vi "Configure Standard Waveform.vi"(8 "error in (no error)":errorcluster, 10 "Std Waveform Setting":T1={"Waveform Function (1: Sine)"=1, "Frequency (1000 Hz)"=1000.0, "Amplitude (1)"=1.0, "Unit (0: Vpp)"=0, "DC Offset (0.00 V)"=0.0} {"Unit (0: Vpp)" items=["Vpp", "Vrms", "dB"]; "Waveform Function (1: Sine)" items=["DC", "Sine", "Square", "Triangle", "Ramp", "Pulse", "Noise", "Sinc", "Negative Ramp", "Exponential Rise", "Exponential Fall", "Cardiac"]}, 11 "Abstract in":refnum<class "Abstract.lvclass">) -> (0 "error out":errorcluster, 3 "Abstract out":refnum<class "Abstract.lvclass">)   [LabVIEW 2016, in "Func Generator.lvlib" / "Abstract.lvclass"]
uses:
  Abstract.lvclass
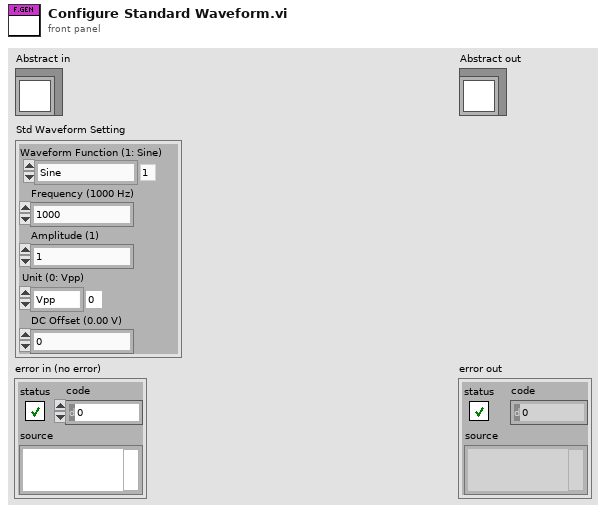
[diagram p1: front panel]
types:
  T1 = cluster{"Waveform Function (1: Sine)":u16, "Frequency (1000 Hz)":dbl, "Amplitude (1)":dbl, "Unit (0: Vpp)":u16, "DC Offset (0.00 V)":dbl}
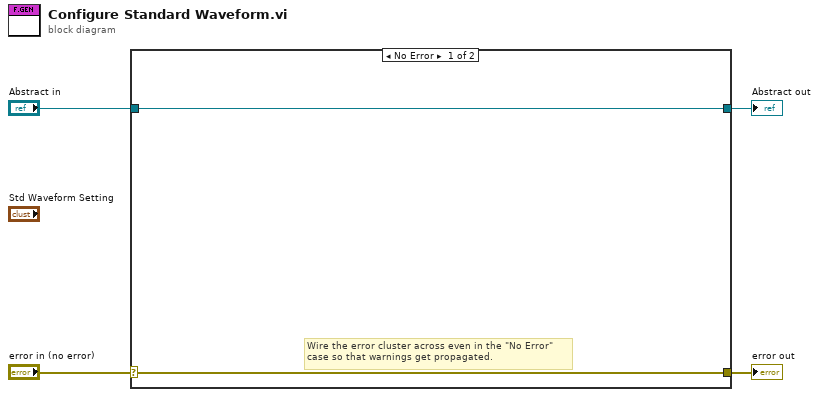
[diagram p0: block diagram]
diagram:
  n1 = case shown="No Error" "error in (no error)" {
    selector: "error in (no error)" -> [w5 w8]
    tunnel: [w5 w8] -> w3
    tunnel: [w6 w7] -> w1
    tunnel: "Abstract in" -> [w6 w7]
    frame No Error {
      # "Wire the error cluster across even in the \"No Error\"\ncase so that warnings get propagated."
    }
    frame Error {
    }
  }
  "error out" <- w3
  "Abstract out" <- w1
